vi "Set Autozero Period.vi"(8 "error in":errorcluster, 10 "Time":u16=10 min=10 max=9999 step=1, 11 "Neph in":refnum<class "Nephelometer.lvclass">) -> (0 "error out":errorcluster, 3 "Neph out":refnum<class "Nephelometer.lvclass">)   [LabVIEW 2014, in "Nephelometer.lvclass"]
uses:
  Nephelometer.lvclass
  Reusable/Session APIs/Serial/Serial Session.lvclass
  Nephelometer.lvclass/Nephelometer.ctl
  Accessors/Read Session Handle.vi
  <userlib>/_Session Fwk/Session - Root.lvclass
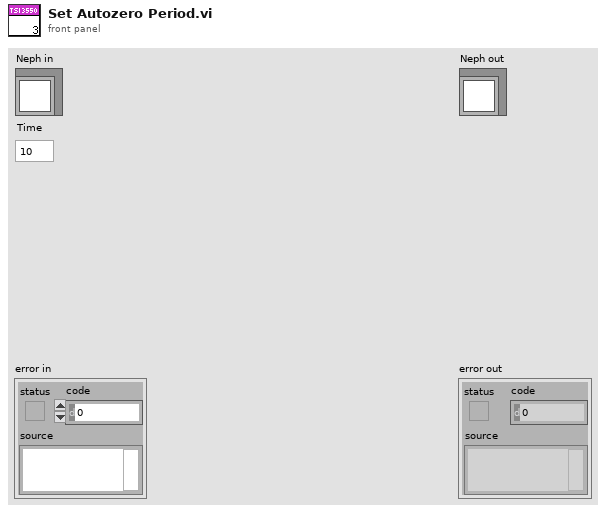
[diagram p1: front panel]
types:
  T1 = typedef "Session - Root.lvclass/Session Handle.ctl" = refnum<data-value>
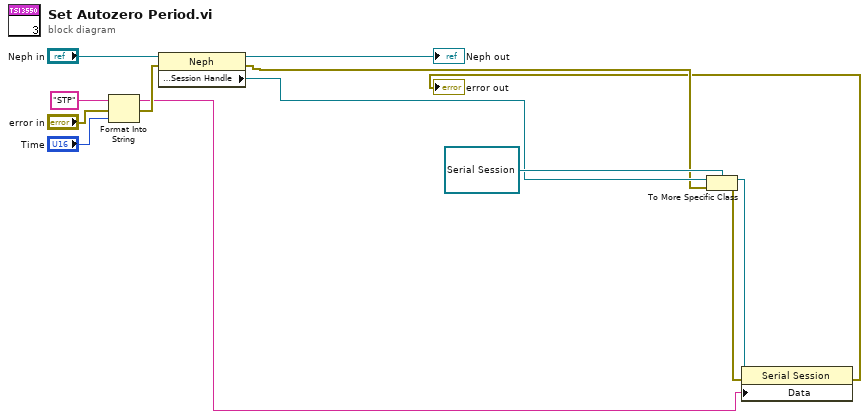
[diagram p0: block diagram]
diagram:
  n1 = Format Into String(initial string="STP", error in="error in", "Time") -> (resulting string=w1:string, error out=w8:errorcluster)  [unwired: 1 in]
  n2 = property class="Neph"(reference="Neph in", error in=w8) -> (reference out=→"Neph out":refnum<class "Nephelometer.lvclass">, error out=w3:errorcluster, "Accessors:Session Handle"=w4:T1)
  n3 = To More Specific Class(target class=refnum<data-value> refnum ("Session Handle"), reference=w4, error in=w3) -> (specific class reference=w6:refnum<data-value>, error out=w5:errorcluster)
  n4 = property class="Serial Session"(reference=w6, error in=w5, "Data"=w1) -> (error out=→"error out":errorcluster)  [unwired: 1 out]
